vi "LimelightDistanceEstimator.vi"() -> ()   [LabVIEW 2017]
uses:
  <vilib>/Rock Robotics/Network Tables/NT Read Number.vi
panel:
  out "Area of Target":dbl
  out "Distance Estimate":dbl
  in  "StopLoop":bool
  in  "TargetHeight":dbl
  in  "CameraHeight":dbl
  in  "CameraAngle":dbl
  # "FIXED CAMERA ANGLE DISTANCE ESTIMATOR"
  # "This will be how far below the horizontal the camera views, since we've put it super high up and angled it down. \nPlease, just keep this number positive, in degrees"
  # "This is in inches. Measure from the floor, to the center of the lense."
  # "This is in inches. Measure from the floor, to the middle of the target (line connecting midpoints of angled tape inner edge)"
  # "If you see an egregious error and need to stop the loop"
  # "Outputted Distance Estimate"
  # "Outputted Area Value"
  # "INSTRUCTIONS:  First off, thank you for helping me out. I know this might be a boring task for you, and its obnoxious that I am not doing it even though this is my project. I've got alot on my plate with this entire thing so this helps me out a bunch. THIS IS AN ABSOLUTELY CRUCIAL ASPECT OF THE PROJECT, so I really appreciate it, and when the robot soars to glory you can take pride in the work you do today. Ok, here's what you need to do, and remember to ask me if something doesn't work and you can't figure it out. Also, please read through this entire thing before you start: Think of this as a really important chemistry lab that requires a good deal of precision.\n\n1) Take Runt, and make sure that camera is mounted and secure. This will not happen immediately on Tuesday, so you may have to do something else in the meantime . . . I may or may not have a task for you . . . I'm sorry for my lack of planning . . . I should have had the camera mounted a while ago . . . ):\n\n2) Once the camera is mounted and secure, measure CameraAngle, CameraHeight, and TargetHeight. Input those into the appropriate boxes, right click, data operations, make current values default. THIS IS AN IMPORTANT STEP\n\n3) Connect to Runt, go to http://limelight.local:5801, and make sure the limelight is tuned (if you don't know how to tune the camera, come get me) and can properly see the target.\n\n4) Verify the code works. If it does not work, see if you can find the error. If you can't come get me. It is working if the run arrow is black and the distance estimate and area of target boxes are not zero. \n\n5) Verify that the distance estimate is reasonable, by using a known distance anc checking against the estimate. If the values are wildly off come get me, cause I probably messed up the math/code.\n\n6) If it giving relatively decent values, then just start logging values in a google sheet. Record actual distance, distance estimate, and area of target. I will draw up the different positions I'd like you to measure from on the whiteboard, or on a piece of paper. I will probably need to be reminded to do this, sorry, I am somewhat forgetful. Finally, if you see a way to improve the code, please feel free to propose the edit to me, or if it common sense and I messed up, just do it. \n\n7) Don't stress about getting all the measurements done today. Try and do as many as you can, but make sure to get any questions in today, since I won't be there Thursday. Again, I really appreciate it, you are doing the team a great service (not to mention yourself)."
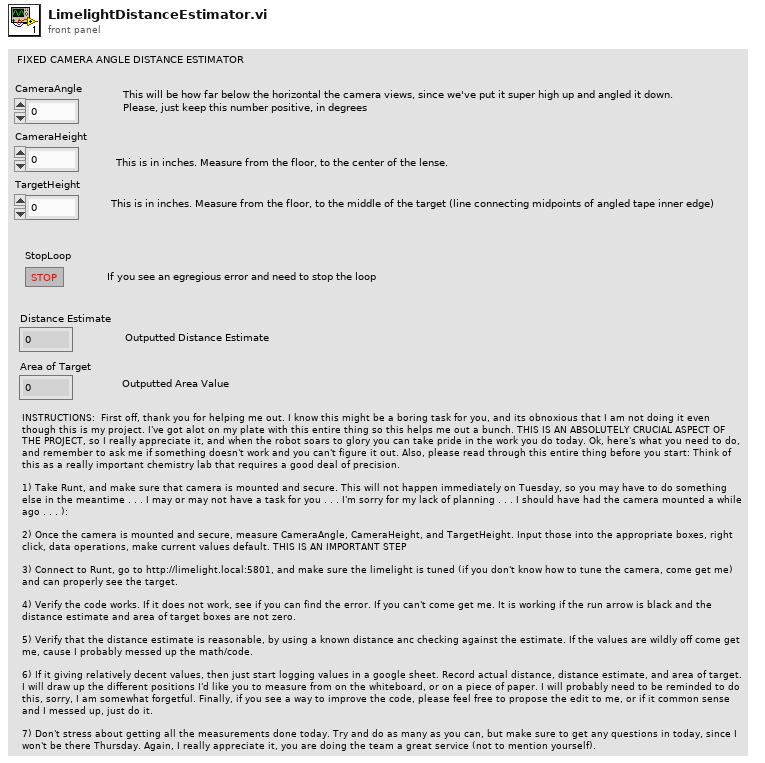
[diagram p1: front panel]
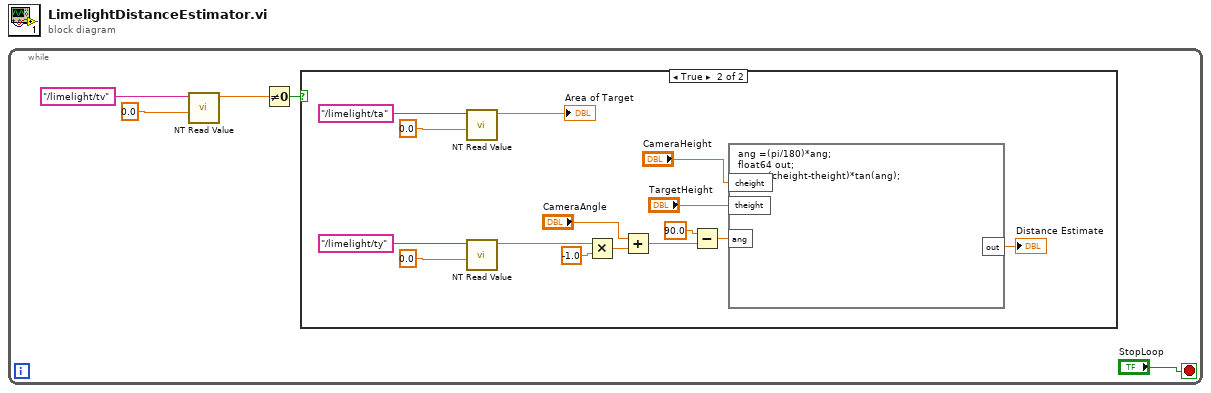
[diagram p0: block diagram]
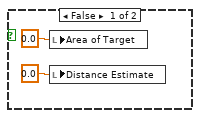
[diagram p2: hidden frame]
diagram:
  n1 = while {
    stop <- "StopLoop" stop-if-true
    n2 = call-poly <vilib>:"NT Read Value.vi"("Default Value"=0.0, "Name"="/limelight/tv") -> ("Numeric"=w2:dbl)  [unwired: 8 in, 1 out]
    n3 = Not Equal To 0?(x=w2) -> (x != 0?=w1:bool)
    n4 = case shown="True" w1 {
      frame False {
        n5 = local write "Area of Target"(0.0 ("Area of Target")) -> ()
        n6 = local write "Distance Estimate"(0.0 ("Distance Estimate")) -> ()
      }
      frame True {
        n7 = call-poly <vilib>:"NT Read Value.vi"("Default Value"=0.0, "Name"="/limelight/ta") -> ("Numeric"=→"Area of Target":dbl)  [unwired: 8 in, 1 out]
        n8 = call-poly <vilib>:"NT Read Value.vi"("Default Value"=0.0, "Name"="/limelight/ty") -> ("Numeric"=w17:dbl)  [unwired: 8 in, 1 out]
        n9 = Multiply(x=w17, y=-1.0) -> (x*y=w16:dbl)
        n10 = Add(x="CameraAngle", y=w16) -> (x+y=w14:dbl)
        n11 = Subtract(x=90.0, y=w14) -> (x-y=w8:dbl)
        n12 = formula code="ang =(pi/180)*ang;\nfloat64 out;\nout = (cheight-theight)*tan(ang);"("cheight"="CameraHeight", "theight"="TargetHeight", "ang"=w8) -> ("out"=→"Distance Estimate":dbl)
      }
    }
  }
